vi "RunningAverage.AddChannels.vi"(8 "Error in":errorcluster, 11 "Waveform Section Refs":T1[](array[typedef]) format="%.0x") -> (0 "Error out":errorcluster)   [LabVIEW 2015, in "Running Average.lvlib"]
uses:
  Running Average.lvlib
  <vilib>/NI Veristand/Custom Device API/Custom Device Item Ref.ctl
  <vilib>/NI Veristand/Custom Device API/Custom Device Channel.ctl
  <vilib>/NI Veristand/Custom Device API/Custom Device Channel Type.ctl
  NationalInstruments.VeriStand.SystemStorage
  Constants.vi
  <vilib>/NI Veristand/Custom Device API/Get Item Property (Dependent Node Pointer).vi
  <vilib>/NI Veristand/Custom Device API/Set Item Property (Dependent Node Pointer).vi
  <vilib>/NI Veristand/Custom Device API/Set Item Property (Double).vi
  <vilib>/NI VeriStand/Custom Device API/Custom Device API.lvlib
  Waveform-Processing-Custom-Device Shared.lvlib
  System Explorer/Waveform-Processing-Custom-Device System Explorer.lvlib
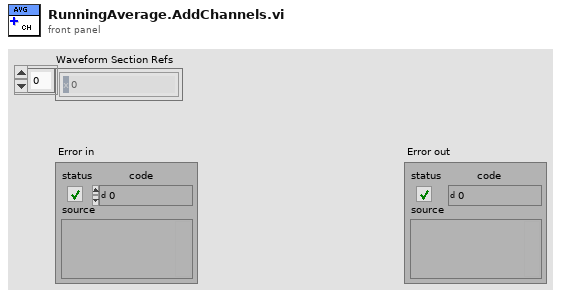
[diagram p1: front panel]
types:
  T1 = typedef "Custom Device API.lvlib/Custom Device Item Ref.ctl" = u64
  T2 = typedef "Custom Device API.lvlib/Custom Device Channel.ctl" = cluster{"Type":T3, "Units":string, "Default Value":dbl, "Faultable":bool, "Scalable":bool}
  T3 = typedef "Custom Device API.lvlib/Custom Device Channel Type.ctl" = enum16{"Input", "Output"}
  T4 = typedef "Custom Device API.lvlib/Custom Device Pointer.ctl" = refnum<k24>
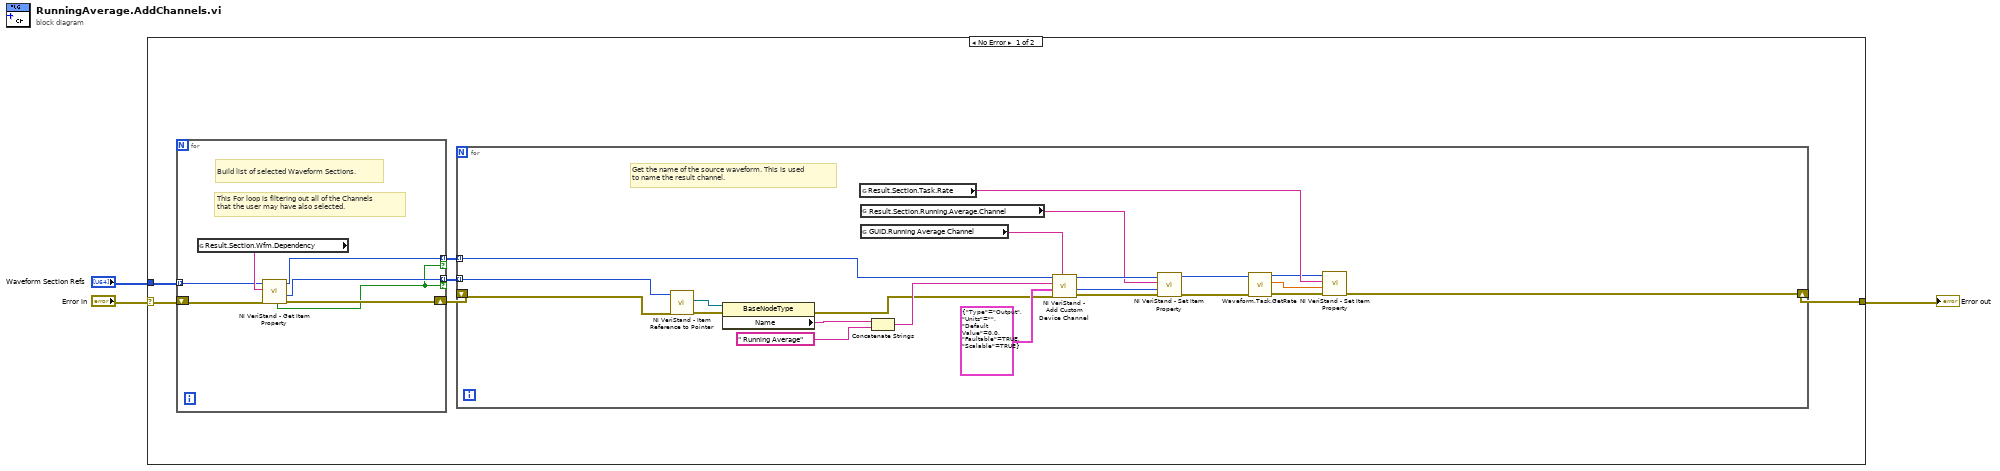
[diagram p0: block diagram]
diagram:
  n1 = case shown="No Error" "Error in" {
    selector: "Error in" -> [w7 w39]
    tunnel: [w9 w39] -> w2
    tunnel: "Waveform Section Refs" -> [w8 _]
    frame No Error {
      n2 = for {
        tunnel: w8 -> [w15] mode=indexing
        shift-right: [w13] -> w6
        shift-left: w7 -> [w14]
        tunnel: [w12] -> w5 mode=indexing if=w10
        tunnel: [w11] -> w4 mode=indexing if=w10
        # "This For loop is filtering out all of the Channels\nthat the user may have also selected."
        # "Build list of selected Waveform Sections."
        n3 = global read "Constants.vi" "Result.Section.Wfm.Dependency"() -> (w16:string)
        n4 = call-poly <vilib>:"NI VeriStand - Get Item Property.vi"("error in (no error)"=w14, "Property Name"=w16, "Item Ref in"=w15) -> ("error out"=w13:errorcluster, "Dependent Node Ref"=w12:T1, "Item Ref out"=w11:T1, "Found"=w10:bool)  [unwired: 5 in]
      }
      n5 = for {
        shift-right: [w17] -> w9
        shift-left: w6 -> [w27]
        tunnel: w5 -> [w26] mode=indexing
        tunnel: w4 -> [w25] mode=indexing
        # "Get the name of the source waveform. This is used\nto name the result channel."
        n6 = call <vilib>:"NI VeriStand - Item Reference to Pointer.vi"("error in (no error)"=w27, "Item Ref in"=w26) -> ("error out"=w36:errorcluster, "Node Pointer"=w32:T4)  [unwired: 6 in, 2 out]
        n7 = property class="BaseNodeType"(reference=w32, error in=w36) -> (error out=w33:errorcluster, "Name"=w35:string)  [unwired: 1 out]
        n8 = global read "Constants.vi" "Result.Section.Task.Rate"() -> (w20:string)
        n9 = global read "Constants.vi" "Result.Section.Running.Average.Channel"() -> (w29:string)
        n10 = global read "Constants.vi" "GUID.Running Average Channel"() -> (w24:string)
        n11 = Concatenate Strings(w35, " Running Average" ("Property Name")) -> (w38:string)
        n12 = call <vilib>:"NI VeriStand - Add Custom Device Channel.vi"("GUID (Default Channel)"=w24, "error in (no error)"=w33, "Channel"=T2 {"Type"=enum."Output", "Units"="", "Default Value"=0.0, "Faultable"=TRUE, "Scalable"=TRUE}, "Channel Name"=w38, "Parent Ref in"=w25) -> ("error out"=w28:errorcluster, "Channel Ref"=w30:T1, "Parent Ref out"=w31:T1)  [unwired: 3 in, 1 out]
        n13 = call-poly <vilib>:"NI VeriStand - Set Item Property.vi"("error in (no error)"=w28, "Dependent Node Ref"=w30, "Property Name"=w29, "Item Ref in"=w31) -> ("error out"=w23:errorcluster, "Item Ref out"=w22:T1)  [unwired: 5 in, 1 out]
        n14 = call "Waveform.Task.GetRate.vi"("error in (no error)"=w23, "Waveform Section Ref in"=w22) -> ("error out"=w19:errorcluster, "Task Rate"=w21:dbl, "Waveform Section Ref out"=w18:T1)  [unwired: 7 in]
        n15 = call-poly <vilib>:"NI VeriStand - Set Item Property.vi"("error in (no error)"=w19, "Value"=w21, "Property Name"=w20, "Item Ref in"=w18) -> ("error out"=w17:errorcluster)  [unwired: 5 in, 2 out]
      }
    }
    frame Error {
    }
  }
  "Error out" <- w2
